vi "NXT_ Init Motor Commands.vi"() -> (0 "_motorCommands":T1)   [LabVIEW 2012, in "Tugboat.lvrbt"]
uses:
  Tugboat.lvrbt
  motorCommands_t.ctl
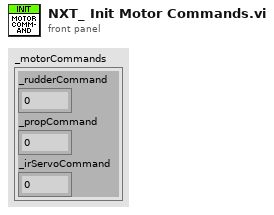
[diagram p1: front panel]
types:
  T1 = typedef "motorCommands_t.ctl" = cluster{"_rudderCommand":i8, "_propCommand":i8, "_irServoCommand":i8}
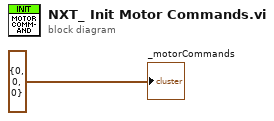
[diagram p0: block diagram]
diagram:
  "_motorCommands" <- T1 {"_rudderCommand"=0, "_propCommand"=0, "_irServoCommand"=0} ("_motorCommands")
